vi "Create Map.vi"(11 "input":string[](array[string])) -> (0 "End":cluster{"row":i32, "col":i32}, 1 "Start":cluster{"row":i32, "col":i32}, 3 "Map":T1(c390), 5 "Heights":i16[][](array[numeric]))   [LabVIEW 2021, in "d12.lvlib"]
uses:
  d12.lvlib
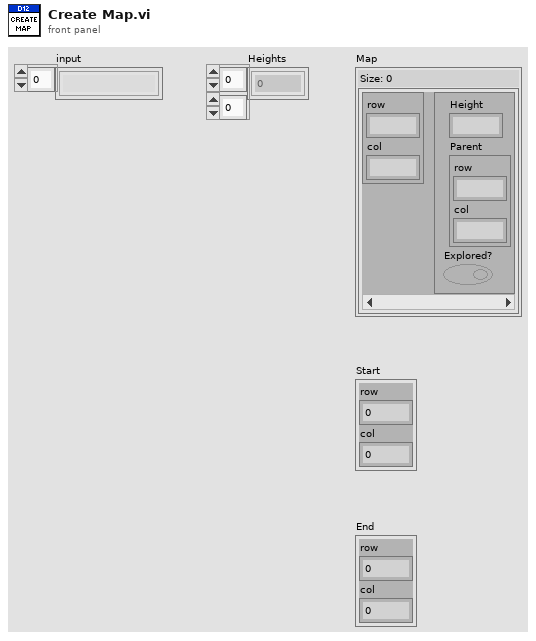
[diagram p1: front panel]
types:
  T1 = map{cluster{"row":i32, "col":i32}, cluster{"Height":i16, "Parent":cluster{"row":i32, "col":i32}, "Explored?":bool}}
  T2 = cluster{"Height":i16, "Parent":cluster{"row":i32, "col":i32}, "Explored?":bool}
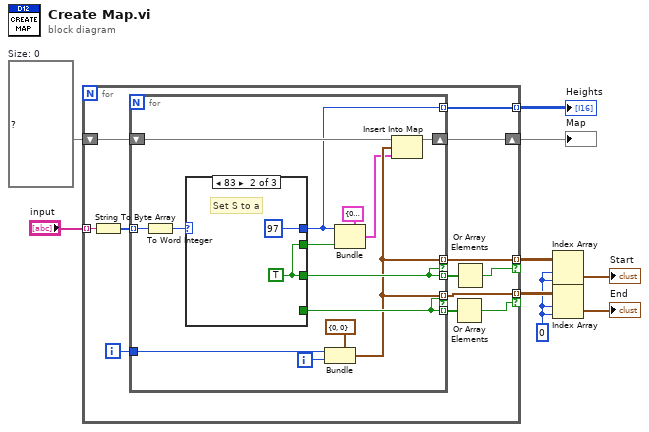
[diagram p0: block diagram]
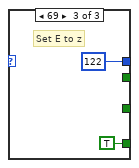
[diagram p3: hidden frame]
diagram:
  w1 = 0 ("index (row)")
  w6 = T1 {}  # Size: 0
  n1 = for {
    tunnel: "input" -> [w21] mode=indexing
    tunnel: [w18] -> w4 mode=indexing if=w16
    tunnel: [w14] -> w5 mode=indexing if=w13
    shift-right: [w12] -> w3
    shift-left: w6 -> [w11]
    tunnel: [w10] -> w9 mode=indexing
    i -> [w19]
    n2 = String To Byte Array(string=w21) -> (unsigned byte array=w20:u8[])
    n3 = for {
      tunnel: w20 -> [w35] mode=indexing
      tunnel: w19 -> [w32]
      tunnel: [w28] -> w18 mode=indexing if=w34
      tunnel: [w34] -> w17 mode=indexing
      tunnel: [w28] -> w14 mode=indexing if=w30
      tunnel: [w30] -> w15 mode=indexing
      shift-right: [w25] -> w12
      shift-left: w11 -> [w26]
      tunnel: [w22] -> w10 mode=indexing
      i -> [w31]
      n4 = To Word Integer(number=w35) -> (16bit integer=w33:i16)
      n5 = case shown="83" w33 {
        selector: w33 -> [w36 _ _]
        tunnel: [w36 i16 97 i16 122] -> w22
        tunnel: [_ w37 _] -> w34
        tunnel: [_ _ TRUE] -> w30
        tunnel: [_ w37 _] -> w24
        frame Default {
        }
        frame 83 {
          w37 = TRUE
          # "Set S to a"
        }
        frame 69 {
          # "Set E to z"
        }
      }
      n6 = Bundle(cluster=cluster{"row":i32, "col":i32} {"row"=0, "col"=0}, "row"=w32, "col"=w31) -> (w28:cluster{"row":i32, "col":i32})
      n7 = Bundle(cluster=T2 {"Height"=0, "Parent"={"row"=0, "col"=0}, "Explored?"=FALSE}, "Height"=w22, "Explored?"=w24) -> (w27:T2)  [unwired: 1 in]
      n8 = Insert Into Map(map in=w26, key=w28, value=w27) -> (map out=w25:T1)  [unwired: 2 out]
    }
    n9 = Or Array Elements(Boolean array=w15) -> (logical OR=w13:bool)
    n10 = Or Array Elements(Boolean array=w17) -> (logical OR=w16:bool)
  }
  "Heights" <- w9
  "Map" <- w3
  n11 = Index Array(array=w4, index (row)=w1, index (col)=w1) -> (element=→"Start":cluster{"row":i32, "col":i32})
  n12 = Index Array(array=w5, index (row)=w1, index (col)=w1) -> (element=→"End":cluster{"row":i32, "col":i32})
